vi "UDP Transmit.vi"(8 "error in (no error)":errorcluster, 9 "Tx":T1, 10 "Transfers":refnum<class "Transfer.lvclass">[](array[class]), 11 "UDP Transceiver in":refnum<class "UDP Transceiver.lvclass">) -> (0 "error out":errorcluster, 3 "UDP Transceiver out":refnum<class "UDP Transceiver.lvclass">)   [LabVIEW 2017, in "UDP.lvlib" / "UDP Transceiver.lvclass"]
uses:
  UDP Transceiver.lvclass
  Builds/Data Sharing Framework/Current/Data Sharing Framework Core/DSF Core.lvlibp/Engine/Classes/Transfer/Transfer.lvclass
  Transfer Group Tx Parameters.ctl
  Transfer Tx Parameters.ctl
  UDP Transceiver.lvclass/UDP Transceiver.ctl
  Builds/Data Sharing Framework/Current/Data Sharing Framework Core/DSF Core.lvlibp/Engine/Classes/Buffer/Buffer.lvclass
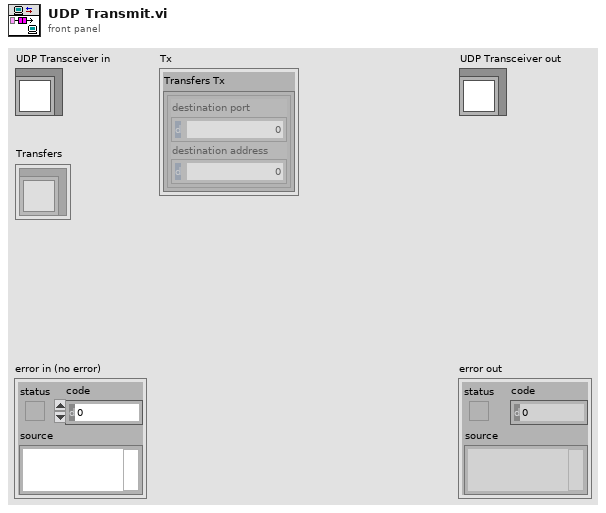
[diagram p1: front panel]
types:
  T1 = typedef "UDP.lvlib/UDP Transceiver.lvclass/Transfer Group Tx Parameters.ctl" = cluster{"Transfers Tx":T2[]}
  T2 = typedef "UDP.lvlib/UDP Transceiver.lvclass/Transfer Tx Parameters.ctl" = cluster{"destination port":u16, "destination address":u32}
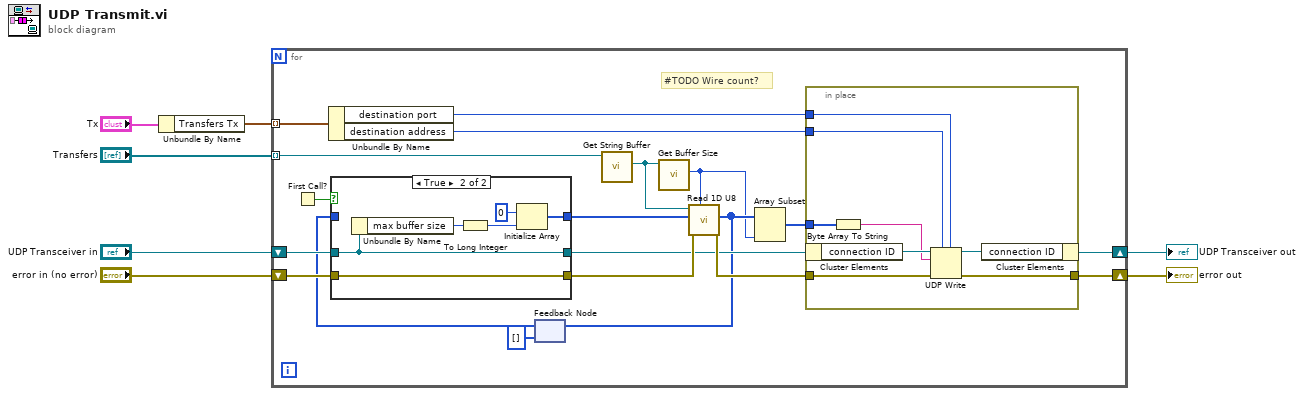
[diagram p0: block diagram]
diagram:
  n1 = Unbundle By Name("Tx") -> ("Transfers Tx"=w7:T2[])
  n2 = for {
    tunnel: "Transfers" -> [w10] mode=indexing
    tunnel: w7 -> [w11] mode=indexing
    shift-right: [w26] -> w4
    shift-left: "error in (no error)" -> [w21]
    shift-right: [w25] -> w3
    shift-left: "UDP Transceiver in" -> [w13]
    # "#TODO Wire count?"
    n3 = First Call?() -> (First Call?: T/F=w18:bool)
    n4 = Unbundle By Name(w11) -> ("destination port"=w23:u16, "destination address"=w24:u32)
    n5 = feedback #1(u8[] [] ("buffer out")) -> (w12:u8[])
    n6 = case shown="True" w18 {
      tunnel: w13 -> [w28 w34]
      tunnel: w21 -> [w29 w35]
      tunnel: [w29 w35] -> w20
      tunnel: [w28 w34] -> w14
      tunnel: w12 -> [w27 _]
      tunnel: [w27 w31] -> w15
      frame False {
      }
      frame True {
        n7 = Unbundle By Name(w34) -> ("max buffer size"=w33:u64)
        n8 = To Long Integer(number=w33) -> (32bit integer=w30:i32)
        n9 = Initialize Array(u8 0 ("element"), w30) -> (w31:u8[])
      }
    }
    n10 = call "Get String Buffer.vi"("Transfer in"=w10) -> ("Buffer"=w19:refnum<class "Buffer.lvclass">)  [unwired: 9 in, 1 out]
    n11 = call "Get Buffer Size.vi"("Buffer in"=w19) -> ("buffer size"=w8:u64)  [unwired: 9 in, 1 out]
    n12 = call "Read 1D U8.vi"("count"=w8, "error in (no error)"=w20, "buffer in"=w15, "Buffer in"=w19) -> ("error out"=w22:errorcluster, "buffer out"=w9:u8[])  [unwired: 4 in, 2 out]
    n13 = feedback-in #1(w9) -> ()
    n14 = Array Subset(array=w9, length=w8) -> (w17:u8[])  [unwired: 1 in]
    n15 = in-place {
      in-place-border: w22 -> [w43]
      in-place-border: [w40] -> w26
      in-place-border: w24 -> [w39]
      in-place-border: w23 -> [w38]
      in-place-border: w17 -> [w37]
      n16 = in-place-cluster #2(w14) -> ("connection ID"=w42:refnum<k16>)
      n17 = Byte Array To String(unsigned byte array=w37) -> (string=w36:string)
      n18 = UDP Write(address=w39, port or service name=w38, connection ID=w42, data in=w36, 8:w43) -> (error out=w40:errorcluster, 3:w41:refnum<k16>)  [unwired: 1 in]
      n19 = in-place-cluster #2("connection ID"=w41) -> (w25:refnum<class "UDP Transceiver.lvclass">)
    }
  }
  "error out" <- w4
  "UDP Transceiver out" <- w3
